vi "生成XY图.vi"(1 "曲线设置":T1={"X轴数据选择"=enum."设置电压", "Y轴组"=[]}, 2 "测试数据":dbl[][](array[numeric])) -> (0 "数组":cluster{"测试数据":dbl[], "测试数据":dbl[]}[](array[cluster]))   [LabVIEW 2021]
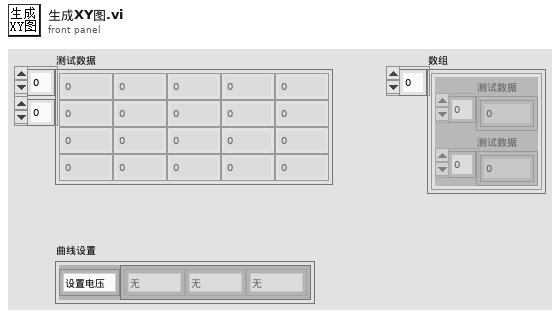
[diagram p1: front panel]
types:
  T1 = typedef "曲线设置.ctl" = cluster{"X轴数据选择":enum16{"时间", "设置电压", "读取电流", "读取电压"}, "Y轴组":enum16{"时间", "设置电压", "读取电流", "读取电压", "无"}[]}
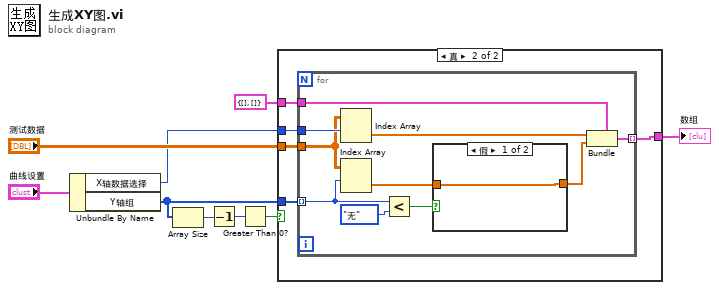
[diagram p0: block diagram]
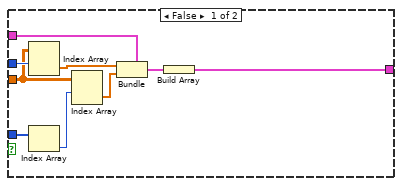
[diagram p2: hidden frame]
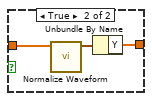
[diagram p3: hidden frame]
diagram:
  n1 = Unbundle By Name("曲线设置") -> ("X轴数据选择"=w7:enum16{"时间", "设置电压", "读取电流", "读取电压"}, "Y轴组"=w5:enum16{"时间", "设置电压", "读取电流", "读取电压", "无"}[])
  n2 = Array Size(array=w5) -> (size(s)=w4:i32)
  n3 = Decrement(x=w4) -> (x-1=w3:i32)
  n4 = Greater Than 0?(x=w3) -> (x > 0?=w2:bool)
  n5 = case shown="真" w2 {
    tunnel: w5 -> [w16 w23]
    tunnel: "测试数据" -> [w17 w22]
    tunnel: w7 -> [w18 w21]
    tunnel: [w10 w20] -> w6
    tunnel: cluster{"X轴":dbl[], "Y轴":dbl[]} {"X轴"=[], "Y轴"=[]} ("簇") -> [w14 w19]
    frame False {
      n6 = Index Array(array=w17, index (row)=w18) -> (element=w13:dbl[])  [unwired: 1 in]
      n7 = Index Array(array=w16) -> (element=w15:enum16{"时间", "设置电压", "读取电流", "读取电压", "无"})  [unwired: 1 in]
      n8 = Index Array(array=w17, index (row)=w15) -> (element=w12:dbl[])  [unwired: 1 in]
      n9 = Bundle(cluster=w14, "X轴"=w13, "Y轴"=w12) -> (w11:cluster{"X轴":dbl[], "Y轴":dbl[]})
      n10 = Build Array(w11) -> (w10:cluster{"X轴":dbl[], "Y轴":dbl[]}[])
    }
    frame True {
      n11 = for {
        tunnel: w23 -> [w26] mode=indexing
        tunnel: w22 -> [w32]
        tunnel: w21 -> [w33]
        tunnel: [w30] -> w20 mode=indexing
        tunnel: w19 -> [w27]
        n12 = Index Array(array=w32, index (row)=w33) -> (element=w31:dbl[])  [unwired: 1 in]
        n13 = Index Array(array=w32, index (row)=w26) -> (element=w29:dbl[])  [unwired: 1 in]
        n14 = Less?(x=w26, y=enum16{"时间", "设置电压", "读取电流", "读取电压", "无"}."无") -> (x < y?=w24:bool)
        n15 = case shown="假" w24 {
          tunnel: w29 -> [w34 w37]
          tunnel: [w34 w35] -> w28
          frame False {
          }
          frame True {
            n16 = call <vilib>:"Normalize Waveform.vi"("waveform in"=w37) -> ("normalized waveform"=w36:waveform(dbl))  [unwired: 7 in, 3 out]
            n17 = Unbundle By Name(w36) -> ("Y"=w35:dbl[])
          }
        }
        n18 = Bundle(cluster=w27, "X轴"=w31, "Y轴"=w28) -> (w30:cluster{"X轴":dbl[], "Y轴":dbl[]})
      }
    }
  }
  "数组" <- w6
